vi "HelloWorld.vi"() -> ()   [LabVIEW 2019]
panel:
  out "Program Output":string
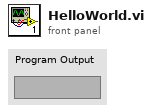
[diagram p1: front panel]
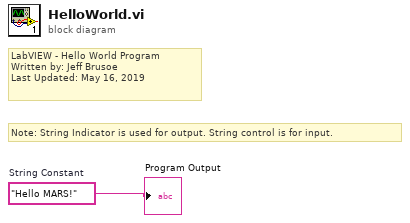
[diagram p0: block diagram]
diagram:
  w1 = "Hello MARS!"  # String Constant
  # "Note: String Indicator is used for output. String control is for input."
  # "LabVIEW - Hello World Program\nWritten by: Jeff Brusoe\nLast Updated: May 16, 2019"
  "Program Output" <- w1
